vi "ORNL DataLogging.vi"() -> ()   [LabVIEW 2016]
panel:
  out "XY Graph":cluster{dbl[], "Filtered X":dbl[]}(graph)
  out "Laser Power":dbl(graph)
  out "Deposition Trigger":bool
  in  "History Data 2":T1(array[cluster])
  in  "History Data":T2(array[cluster])
  out "Pyrometer Measurements":T3(graph)
  in  "Pyrometer Names":string[](array[string])=["MI-18", "M322"]
  out "Data Path":path=path "C:/Users/Mark/Documents/GKN Instrumentation and Control/Data/Build Data Mon Oct 02, 2017 14_52_50  "
  in  "Write Data to File":bool
  out "TC Measurements":T4(graph)
  in  "ABORT":bool
  in  "TC Names":string[](array[string])=["Nozzle", "Copper Plate", "Aluminum Cooling Block", "Bottom Downtube", "Coverslide Module", "Free Floating", "Camera", "Optics", "T-BP-0", "T-BP-1", "T-BP-2", "T-BP-3", "T-BP-4", "T-BP-5", "T-BP-6", "T-BP-7", "T-BP-8", "T-MP-0", "T-MP-1", "T-MP-2", "T-MP-3", "T-MP-4", "T-MP-5", "T-MP-6", "T-AT-0", "T-AT-1", "T-AT-2", "T-AT-3", "T-AT-4", "T-AT-5", "T-CL-0", "T-SB-0"]
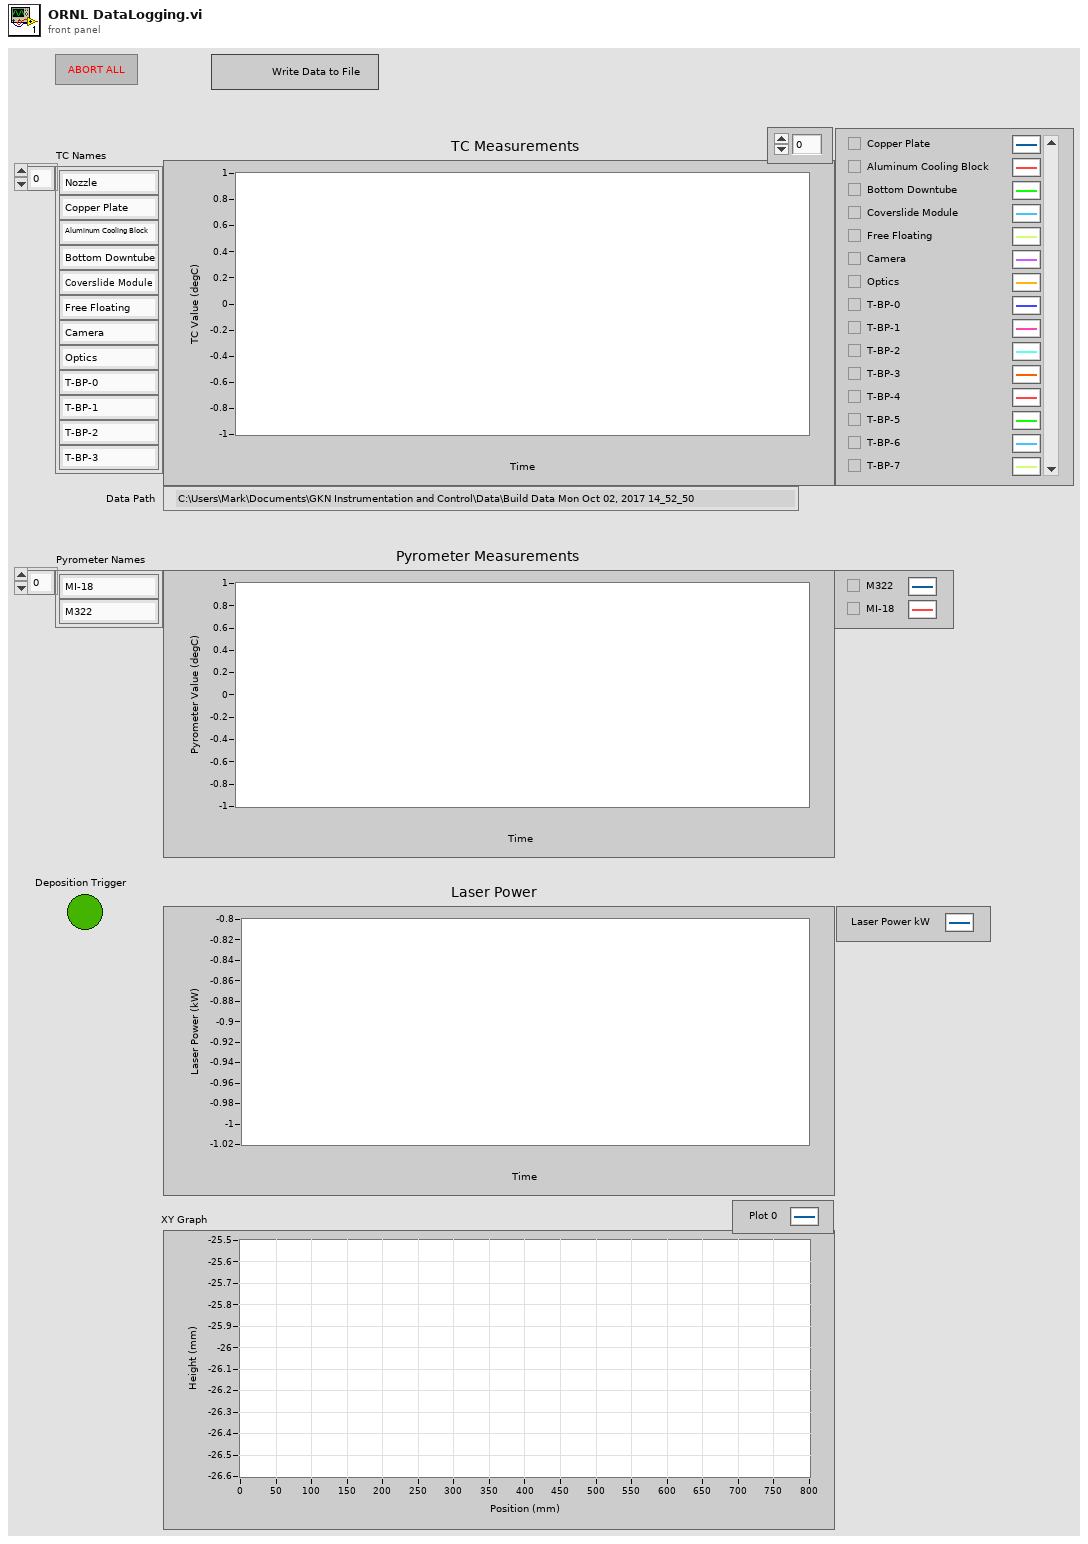
[diagram p1: front panel]
types:
  T1 = cluster{"Array of Double[0]":dbl, "Array of Double[1]":dbl}[]
  T2 = cluster{"Array of Double[0]":dbl, "Array of Double[1]":dbl, "Array of Double[2]":dbl, "Array of Double[3]":dbl, "Array of Double[4]":dbl, "Array of Double[5]":dbl, "Array of Double[6]":dbl, "Array of Double[7]":dbl, "Array of Double[8]":dbl, "Array of Double[9]":dbl, "Array of Double[10]":dbl, "Array of Double[11]":dbl, "Array of Double[12]":dbl, "Array of Double[13]":dbl, "Array of Double[14]":dbl, "Array of Double[15]":dbl, "Array of Double[16]":dbl, "Array of Double[17]":dbl, "Array of Double[18]":dbl, "Array of Double[19]":dbl, "Array of Double[20]":dbl, "Array of Double[21]":dbl, "Array of Double[22]":dbl, "Array of Double[23]":dbl, "Array of Double[24]":dbl, "Array of Double[25]":dbl, "Array of Double[26]":dbl, "Array of Double[27]":dbl, "Array of Double[28]":dbl, "Array of Double[29]":dbl, "Array of Double[30]":dbl, "Array of Double[31]":dbl}[]
  T3 = cluster{"Array of Double[0]":dbl, "Array of Double[1]":dbl}
  T4 = cluster{"Array of Double[0]":dbl, "Array of Double[1]":dbl, "Array of Double[2]":dbl, "Array of Double[3]":dbl, "Array of Double[4]":dbl, "Array of Double[5]":dbl, "Array of Double[6]":dbl, "Array of Double[7]":dbl, "Array of Double[8]":dbl, "Array of Double[9]":dbl, "Array of Double[10]":dbl, "Array of Double[11]":dbl, "Array of Double[12]":dbl, "Array of Double[13]":dbl, "Array of Double[14]":dbl, "Array of Double[15]":dbl, "Array of Double[16]":dbl, "Array of Double[17]":dbl, "Array of Double[18]":dbl, "Array of Double[19]":dbl, "Array of Double[20]":dbl, "Array of Double[21]":dbl, "Array of Double[22]":dbl, "Array of Double[23]":dbl, "Array of Double[24]":dbl, "Array of Double[25]":dbl, "Array of Double[26]":dbl, "Array of Double[27]":dbl, "Array of Double[28]":dbl, "Array of Double[29]":dbl, "Array of Double[30]":dbl, "Array of Double[31]":dbl}
  T5 = enum16{"open", "open or create", "create or replace", "create", "open (read-only)"}
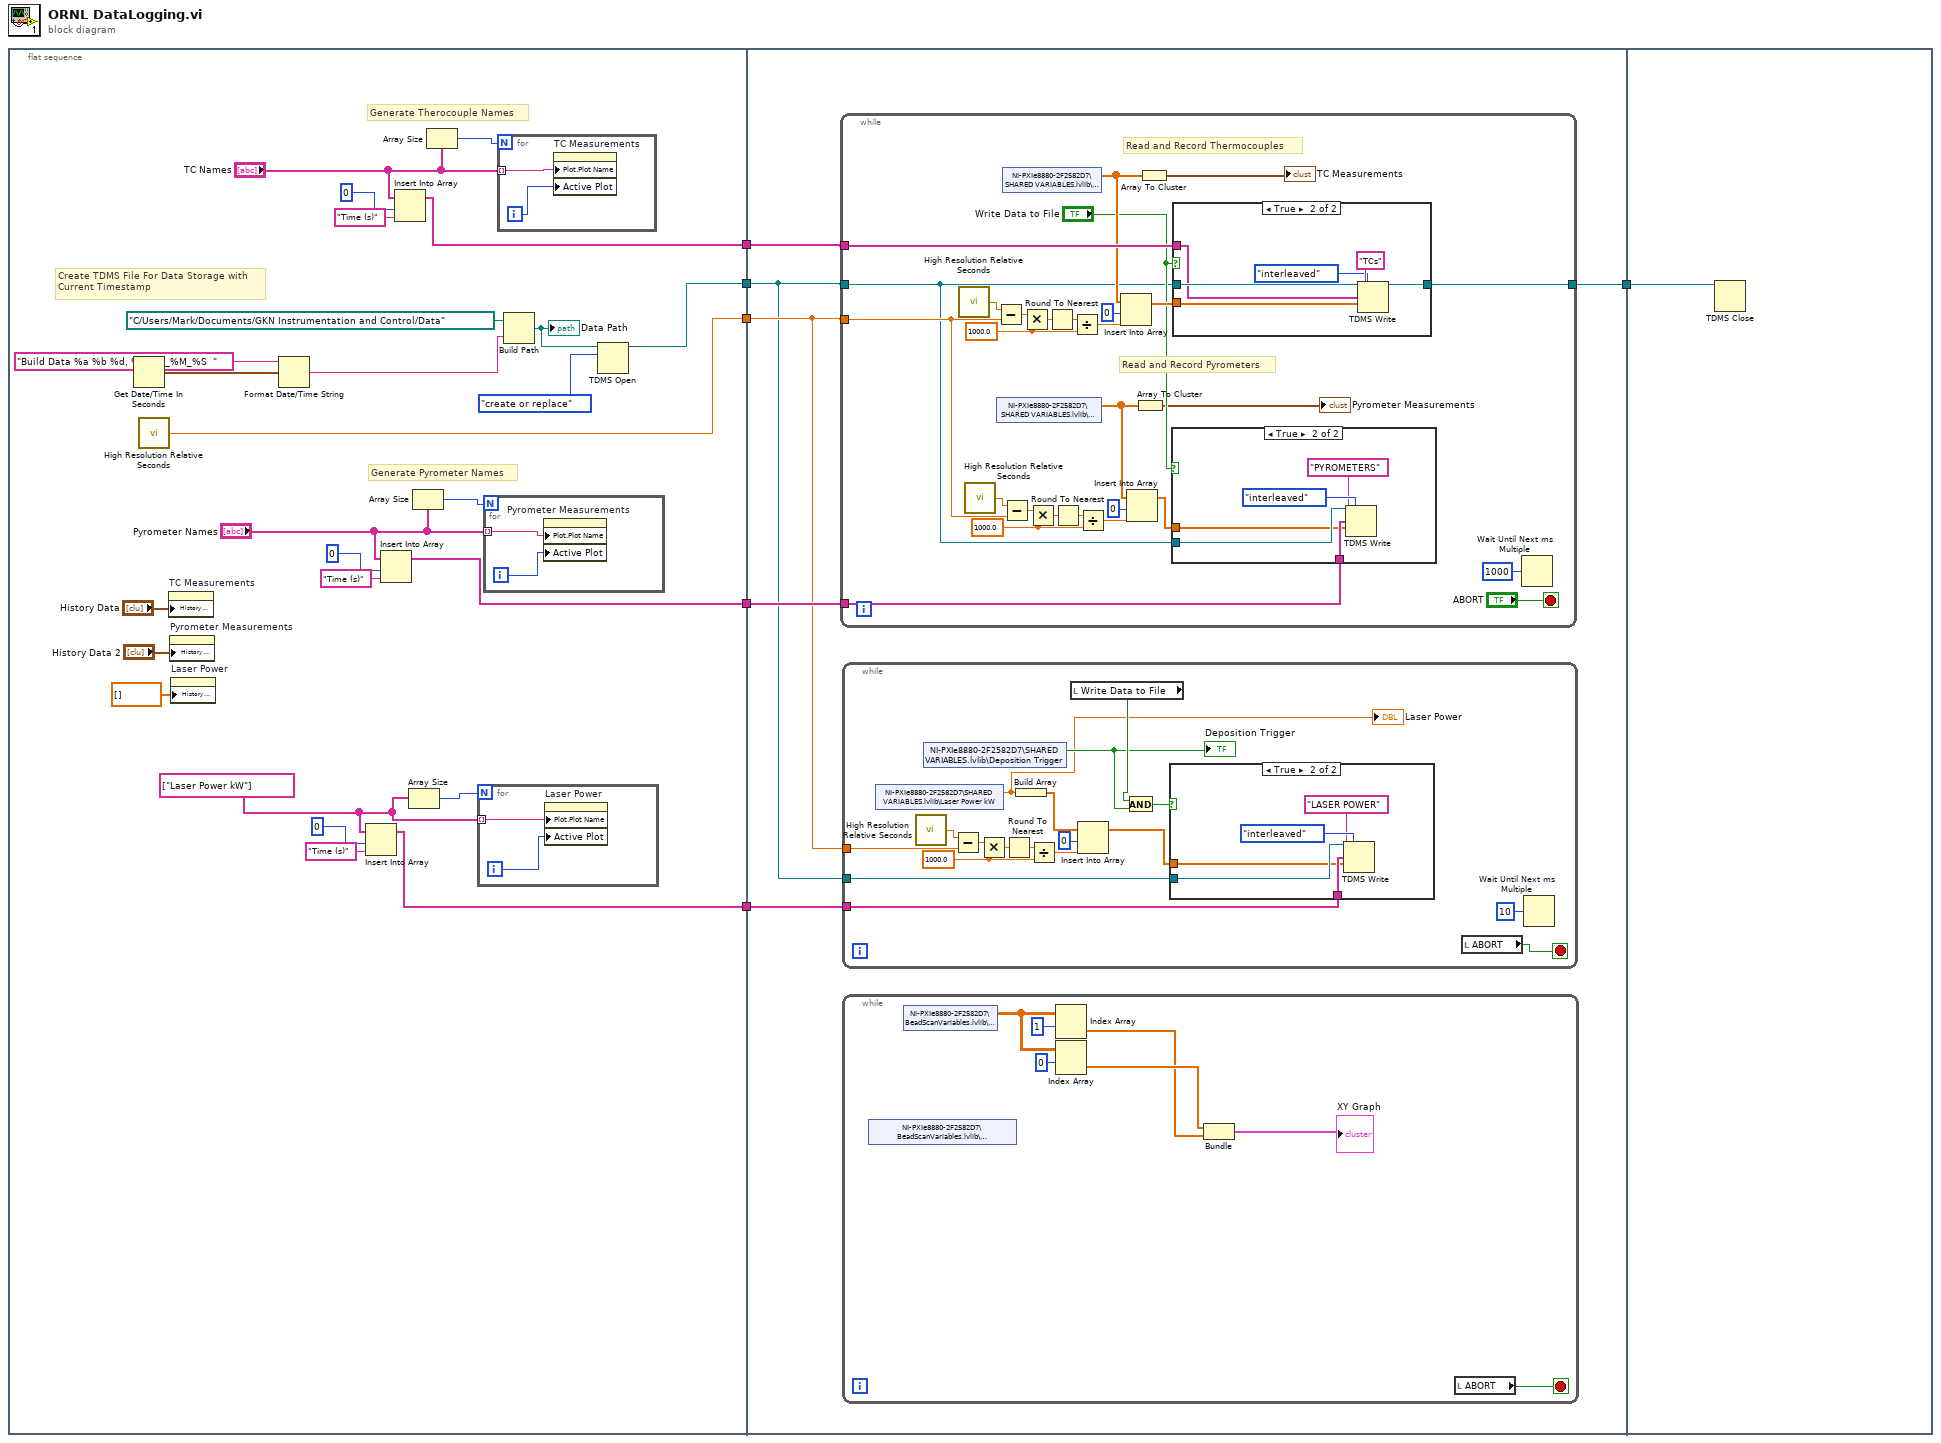
[diagram p0: block diagram]
diagram:
  n1 = flat-sequence {
    tunnel: [w25] -> w6
    tunnel: [w21] -> w5
    tunnel: [w20] -> w4
    tunnel: [w15] -> w3
    tunnel: [w9] -> w1
    tunnel: w6 -> [w40]
    tunnel: w5 -> [w44]
    tunnel: w4 -> [w41]
    tunnel: w3 -> [w43]
    tunnel: [w42] -> w2
    tunnel: w1 -> [w39]
    tunnel: w2 -> [w115]
    frame #0 {
      w8 = string[] ["Laser Power kW"]
      # "Create TDMS File For Data Storage with\nCurrent Timestamp"
      # "Generate Pyrometer Names"
      # "Generate Therocouple Names"
      n2 = Get Date/Time In Seconds() -> (seconds since 1Jan1904=w30:timestamp)
      n3 = call <vilib>:"High Resolution Relative Seconds.vi"() -> ("relative seconds"=w20:dbl)
      n4 = property on="TC Measurements" class="WFChart (strict)"("History Data"="History Data") -> ()  [unwired: 2 in, 2 out]
      n5 = property on="Pyrometer Measurements" class="WFChart (strict)"("History Data"="History Data 2") -> ()  [unwired: 2 in, 2 out]
      n6 = property on="Laser Power" class="WFChart (strict)"("History Data"=dbl[] []) -> ()  [unwired: 2 in, 2 out]
      n7 = Format Date/Time String(time format string (%c)="Build Data %a %b %d, %Y %H_%M_%S  ", seconds (now)=w30) -> (date/time string=w28:string)  [unwired: 1 in]
      n8 = Insert Into Array(array=w8, index=0, new element="Time (s)" ("new element/subarray")) -> (w9:string[])
      n9 = Insert Into Array(array="Pyrometer Names", index=0, new element="Time (s)" ("new element/subarray")) -> (w15:string[])
      n10 = Insert Into Array(array="TC Names", index=0, new element="Time (s)" ("new element/subarray")) -> (w21:string[])
      n11 = Array Size(array=w8) -> (size(s)=w10:i32)
      n12 = Array Size(array="Pyrometer Names") -> (size(s)=w19:i32)
      n13 = Array Size(array="TC Names") -> (size(s)=w32:i32)
      n14 = for {
        N: w10 -> [_]
        tunnel: w8 -> [w34] mode=indexing
        i -> [w33]
        n15 = property on="Laser Power" class="WFChart (strict)"("Plot.Plot Name"=w34, "Active Plot"=w33) -> ()  [unwired: 2 in, 2 out]
      }
      n16 = for {
        N: w19 -> [_]
        tunnel: "Pyrometer Names" -> [w36] mode=indexing
        i -> [w35]
        n17 = property on="Pyrometer Measurements" class="WFChart (strict)"("Plot.Plot Name"=w36, "Active Plot"=w35) -> ()  [unwired: 2 in, 2 out]
      }
      n18 = for {
        N: w32 -> [_]
        tunnel: "TC Names" -> [w37] mode=indexing
        i -> [w38]
        n19 = property on="TC Measurements" class="WFChart (strict)"("Plot.Plot Name"=w37, "Active Plot"=w38) -> ()  [unwired: 2 in, 2 out]
      }
      n20 = Build Path(base path=path "C:/Users/Mark/Documents/GKN Instrumentation and Control/Data", name or relative path=w28) -> (appended path=w27:path)
      "Data Path" <- w27
      n21 = TDMS Open(10:T5."create or replace" ("operation (0:open)"), 11:w27) -> (3:w25:refnum<k34>)  [unwired: 5 in, 1 out]
    }
    frame #1 {
      n22 = while {
        tunnel: w40 -> [w78]
        tunnel: [w99] -> w42
        tunnel: w44 -> [w98]
        tunnel: w41 -> [w81]
        tunnel: w43 -> [w77]
        stop <- "ABORT" stop-if-true
        w83 = 1000.0 ("y")
        w90 = 1000.0 ("y")
        # "Read and Record Pyrometers"
        # "Read and Record Thermocouples"
        n23 = call <vilib>:"High Resolution Relative Seconds.vi"() -> ("relative seconds"=w97:dbl)
        n24 = call <vilib>:"High Resolution Relative Seconds.vi"() -> ("relative seconds"=w88:dbl)
        n25 = Subtract(x=w97, y=w81) -> (x-y=w93:dbl)
        n26 = shared-variable "NI-PXIe8880-2F2582D7\\SHARED VARIABLES.lvlib\\Pyrometers"() -> (w80:dbl[])  [unwired: 1 in, 1 out]
        n27 = Subtract(x=w88, y=w81) -> (x-y=w86:dbl)
        n28 = shared-variable "NI-PXIe8880-2F2582D7\\SHARED VARIABLES.lvlib\\TC's Array"() -> (w96:dbl[])  [unwired: 1 in, 1 out]
        n29 = Multiply(x=w93, y=w90) -> (x*y=w92:dbl)
        n30 = Multiply(x=w86, y=w83) -> (x*y=w85:dbl)
        n31 = Round To Nearest(number=w92) -> (nearest integer value=w91:dbl)
        n32 = Round To Nearest(number=w85) -> (nearest integer value=w84:dbl)
        n33 = Divide(x=w91, y=w90) -> (x/y=w89:dbl)
        n34 = Divide(x=w84, y=w83) -> (x/y=w82:dbl)
        n35 = Insert Into Array(array=w96, index=0, new element=w89) -> (w94:dbl[])
        n36 = Insert Into Array(array=w80, index=0, new element=w82) -> (w76:dbl[])
        n37 = Array To Cluster(array=w80) -> (cluster=→"Pyrometer Measurements":T3)
        n38 = Array To Cluster(array=w96) -> (cluster=→"TC Measurements":T4)
        n39 = case shown="True" "Write Data to File" {
          tunnel: w78 -> [_ w105]
          tunnel: w77 -> [_ w104]
          tunnel: w76 -> [_ w103]
          frame False {
          }
          frame True {
            n40 = TDMS Write(0:w105, 1:enum16{"decimated", "interleaved"}."interleaved" ("data layout (0:decimated)"), 5:"PYROMETERS" ("group name in (Untitled)"), 7:w104, 9:w103) -> ()  [unwired: 1 in, 4 out]
          }
        }
        n41 = case shown="True" "Write Data to File" {
          tunnel: w78 -> [w108 w114]
          tunnel: w98 -> [_ w110]
          tunnel: [w108 w113] -> w99
          tunnel: w94 -> [_ w109]
          frame False {
          }
          frame True {
            n42 = TDMS Write(0:w114, 1:enum16{"decimated", "interleaved"}."interleaved" ("data layout (0:decimated)"), 5:"TCs" ("group name in (Untitled)"), 7:w110, 9:w109) -> (4:w113:refnum<k34>)  [unwired: 1 in, 3 out]
          }
        }
        n43 = Wait Until Next ms Multiple(millisecond multiple=u32 1000) -> ()  [unwired: 1 out]
      }
      n44 = while {
        tunnel: w41 -> [w61]
        tunnel: w40 -> [w58]
        tunnel: w39 -> [w57]
        stop <- w52 stop-if-true
        w63 = 1000.0 ("y")
        n45 = shared-variable "NI-PXIe8880-2F2582D7\\SHARED VARIABLES.lvlib\\Laser Power kW"() -> (w53:dbl)  [unwired: 1 in, 1 out]
        "Laser Power" <- w53
        n46 = call <vilib>:"High Resolution Relative Seconds.vi"() -> ("relative seconds"=w68:dbl)
        n47 = shared-variable "NI-PXIe8880-2F2582D7\\SHARED VARIABLES.lvlib\\Deposition Trigger"() -> (w54:bool)  [unwired: 1 in, 1 out]
        "Deposition Trigger" <- w54
        n48 = Subtract(x=w68, y=w61) -> (x-y=w66:dbl)
        n49 = Multiply(x=w66, y=w63) -> (x*y=w65:dbl)
        n50 = Round To Nearest(number=w65) -> (nearest integer value=w64:dbl)
        n51 = Build Array(w53) -> (w60:dbl[])
        n52 = Divide(x=w64, y=w63) -> (x/y=w62:dbl)
        n53 = local read "Write Data to File"() -> (w55:bool)
        n54 = Insert Into Array(array=w60, index=0, new element=w62) -> (w59:dbl[])
        n55 = And(x=w55, y=w54) -> (x .and. y?=w56:bool)
        n56 = case shown="True" w56 {
          tunnel: w58 -> [_ w72]
          tunnel: w57 -> [_ w71]
          tunnel: w59 -> [_ w70]
          frame False {
          }
          frame True {
            n57 = TDMS Write(0:w72, 1:enum16{"decimated", "interleaved"}."interleaved" ("data layout (0:decimated)"), 5:"LASER POWER" ("group name in (Untitled)"), 7:w71, 9:w70) -> ()  [unwired: 1 in, 4 out]
          }
        }
        n58 = local read "ABORT"() -> (w52:bool)
        n59 = Wait Until Next ms Multiple(millisecond multiple=u32 10) -> ()  [unwired: 1 out]
      }
      n60 = while {
        stop <- w46 stop-if-true
        n61 = shared-variable "NI-PXIe8880-2F2582D7\\BeadScanVariables.lvlib\\BeadScanComplete"() -> ()  [unwired: 1 in, 2 out]
        n62 = shared-variable "NI-PXIe8880-2F2582D7\\BeadScanVariables.lvlib\\ScanData"() -> (w50:dbl[][])  [unwired: 1 in, 1 out]
        n63 = Index Array(array=w50, index (row)=1) -> (element=w45:dbl[])  [unwired: 1 in]
        n64 = Index Array(array=w50, index (row)=0) -> (element=w48:dbl[])  [unwired: 1 in]
        n65 = Bundle(w48, w45) -> (→"XY Graph":cluster{dbl[], dbl[]})  [unwired: 1 in]
        n66 = local read "ABORT"() -> (w46:bool)
      }
    }
    frame #2 {
      n67 = TDMS Close(11:w115) -> ()  [unwired: 1 in, 2 out]
    }
  }
